vi "运维调试_采配水.vi"() -> ()   [LabVIEW 2016, in "PLC.lvlib"]
uses:
  PLC.lvlib
  <vilib>/Plasmionique/MB Master/MB_Master/MB_Master.lvclass
  <vilib>/Utility/miscctls.llb/LVPointTypeDef.ctl
  <vilib>/Plasmionique/MB Master/MB_Master_Serial/MB_Master_Serial.lvclass
  C:/Program Files (x86)/National Instruments/LabVIEW 2016/vi.lib/Plasmionique/MB Master/MB_Master/MB_Master.lvclass
  <vilib>/Plasmionique/MB Master/MB Master.lvlib
panel:
  in  "是否启用质控":u16(ring) items=["不启用质控", "启用质控"]
  out "压力传感器":dbl format="%#.2f"
  out "R110":i16 caption="过滤装置排液时间"
  out "X12":bool caption="过滤溢流液位开关"
  in  "M4":bool
  in  "M3":bool
  in  "V14NC":bool
  in  "V14NO":bool
  in  "V13NC":bool
  in  "V13NO":bool
  in  "V12":bool
  in  "V11":bool
  in  "V10":bool
  in  "V9":bool
  in  "V8":bool
  in  "V7NC":bool
  in  "V7NO":bool
  out "R113":i16 caption="反冲洗排液时间"
  out "X2":bool caption="X1"
  out "采配水版本号":string
  out "R23":i16 caption="清洗频次计数"
  out "R112":i16 caption="清洗频次设定"
  out "R111":i16 caption="排液时间"
  out "通讯故障":bool
  in  "潜水泵工作模式":u16(ring) items=["泵1单泵单管路", "泵2单泵单管路", "双泵双管路"]
  out "X11":bool caption="自来水检测"
  out "X10":bool caption="空压机压力报警"
  out "X9":bool caption="废液报警"
  out "X8":bool caption="泵2过载报警"
  out "X7":bool caption="泵1过载报警"
  out "X6":bool caption="断电检测"
  out "X5":bool caption="开门检测"
  out "X4":bool caption="烟雾检测"
  out "X3":bool caption="漏水检测"
  out "X1":bool
  out "X0":bool caption="采样池液位开关"
  out "R109":i16 caption="外部反冲洗时间"
  out "集成报警信息":string
  out "R108":i16 caption="进样超时时间"
  out "R107":i16 caption="进气时间"
  out "R106":i16 caption="反冲洗排液时间"
  out "R105":i16 caption="配水时间"
  out "R104":i16 caption="过滤次数"
  out "R103":i16 caption="过滤配水时间"
  out "R102":i16 caption="静置沉淀时间"
  out "R101":i16 caption="管路润洗时间"
  out "R100":i16 caption="外部管路润洗时间"
  out "R2":i16
  out "R1":i16
  out "多列列表框":i32(listbox)
  in  "V6":bool
  in  "V5":bool
  in  "V4":bool
  in  "V3":bool
  in  "V2":bool
  in  "M2":bool
  in  "V1":bool
  in  "M1":bool
  in  "返回":bool
  in  "参数设置":bool
  in  "单步启动":bool
  in  "启动":bool
  in  "停止":bool
  # "流程计时："
  # "s"
  # "压力传感器："
  # "MPa"
  # "二级液位开关低"
  # "二级液位开关高"
  # "次"
  # "S"
  # "S"
  # "次"
  # "次"
  # "S"
  # "S"
  # "S"
  # "S"
  # "S"
  # "S"
  # "S"
  # "S"
  # "S"
  # "单步计时："
  # "s"
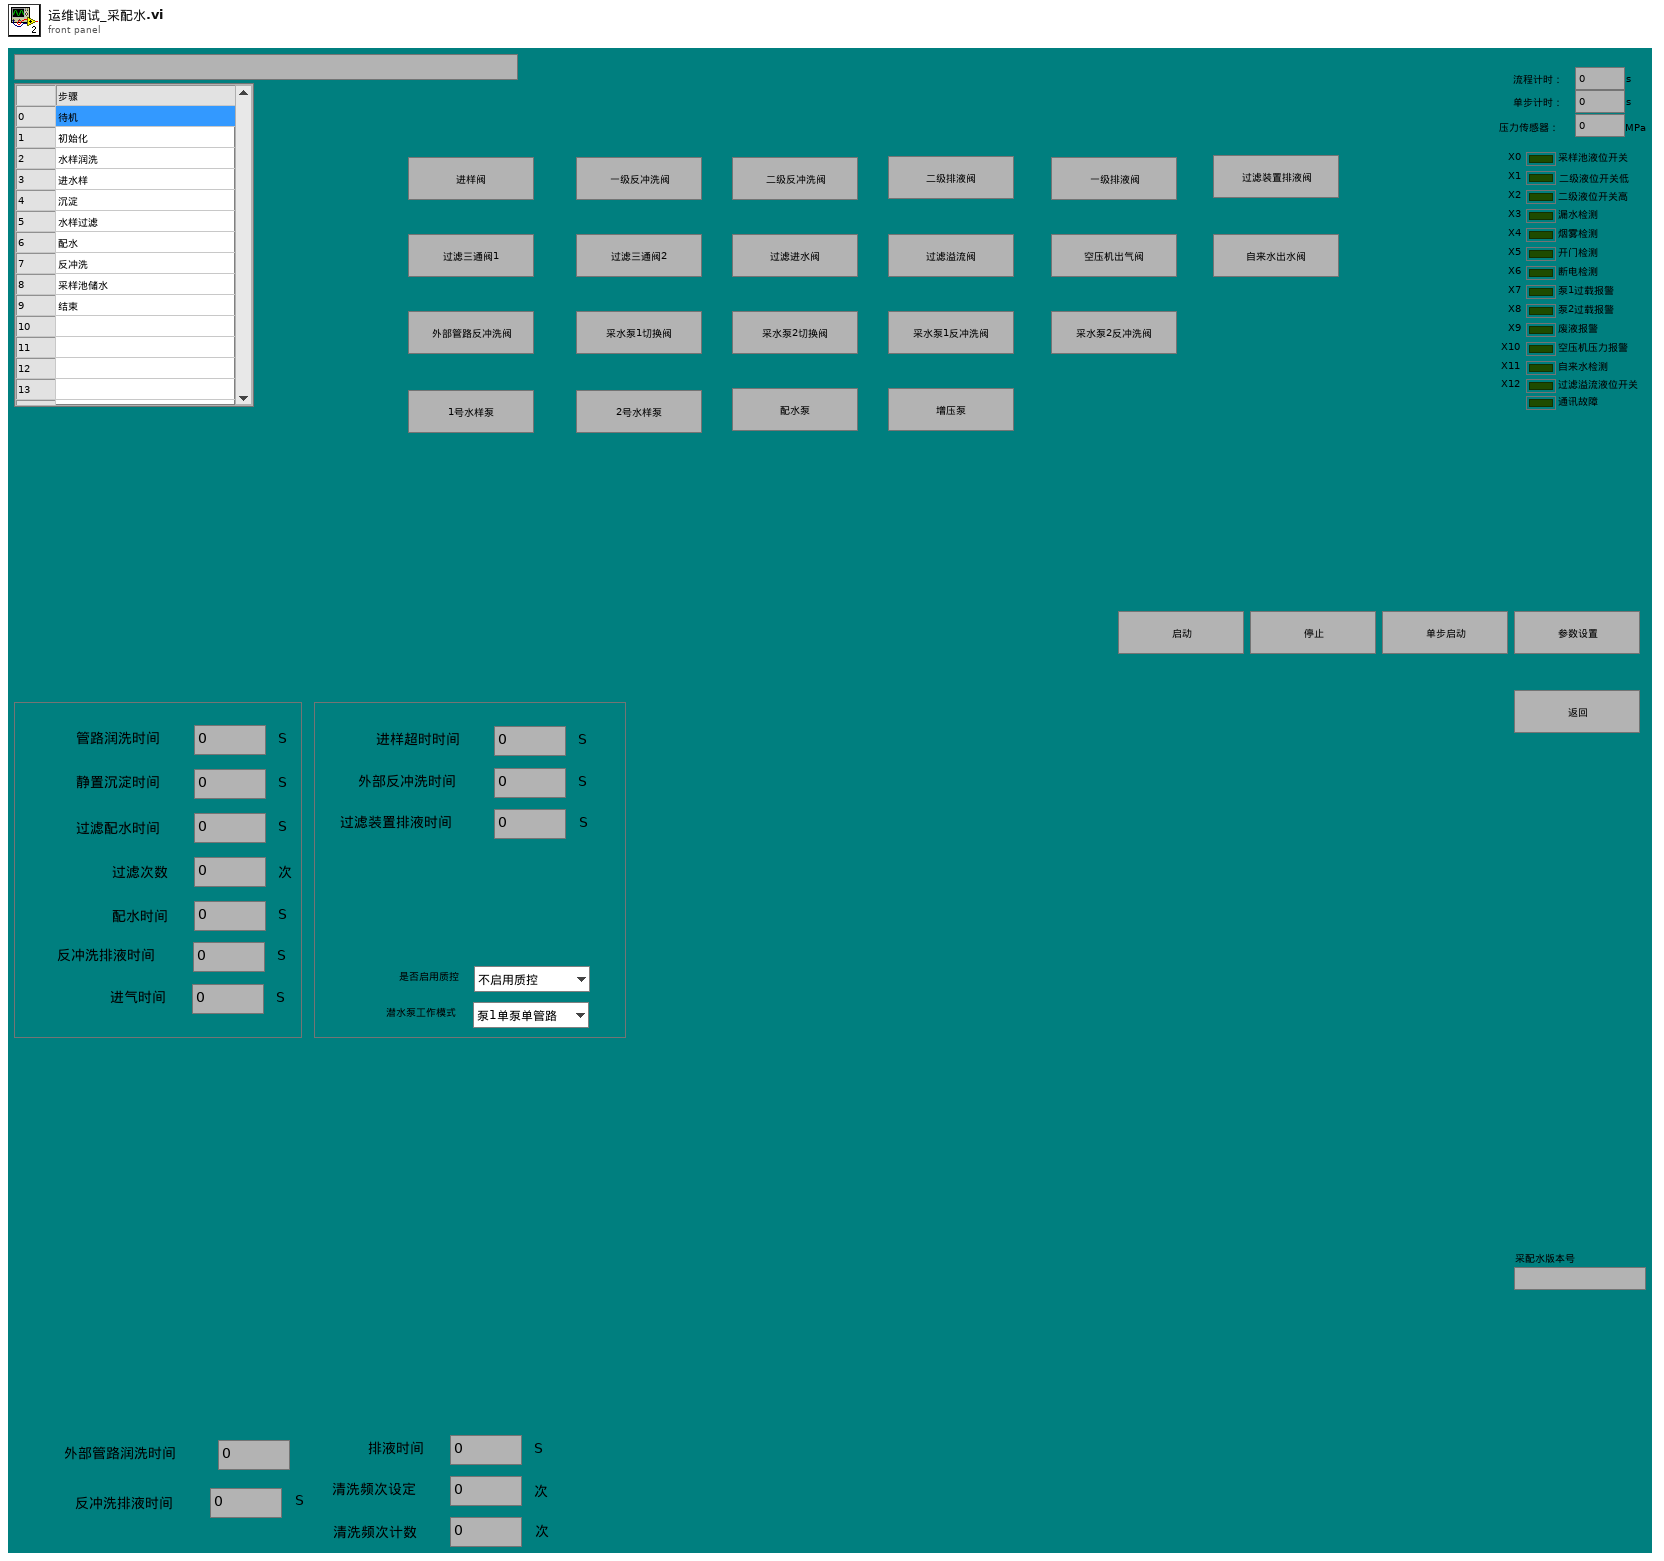
[diagram p1: front panel]
types:
  T1 = typedef "LVPointTypeDef.ctl" = cluster{"Horizontal":i16, "Vertical":i16}
  T2 = cluster{"时间标识":timestamp, "设备":string, "日志信息":string}
  T3 = cluster{"R0":i16, "R1":i16, "R2":i16, "R3":i16, "R4":i16, "R5":i16, "R6":i16, "R7":i16, "R8":i16, "R9":i16, "R10":i16, "R11":i16, "R12":i16, "R13":i16, "R14":i16, "R15":i16, "R16":i16, "R17":i16, "R18":i16, "R19":i16, "R20":i16, "R21":i16, "R22":i16, "R23":i16, "R24":i16, "R25":i16}
  T4 = cluster{"seconds since 1Jan1904":timestamp, "table输入":string, string, "table输入":string}
  T5 = cluster{"时间标识":timestamp, "设备":string, "日志信息":string, "流程参数":string}
  T6 = cluster{"命令":string, cluster{"starting address":u16, "holding register value":u16}}
  T7 = cluster{"CODCr":cluster{"启动测量模式":cluster{"测量模式":enum16{"水样测量", "标样核查", "零点核查", "加标回收", "平行样", "校零", "校标"}}, "确定按钮":bool}, "参数启用":cluster{"多参数":bool, "CODMn":bool, "总磷总氮":bool, "氨氮":bool, "CODcr":bool}}
  T8 = enum16{"水样测量", "标样核查", "零点核查", "加标回收", "平行样", "校零", "校标"}
  T9 = cluster{"命令":string, "数据":cluster{"starting address":u16, "holding register value":u16}}
  T10 = cluster{"命令":string, "数据":cluster{"starting address":u16, "holding register values":u16[]}}
  T11 = cluster{"命令":string, "data":cluster{"starting address":u16, "coil values":bool[]}}
  T12 = cluster{"多参数":bool, "CODMn":bool, "总磷总氮":bool, "氨氮":bool, "CODcr":bool}
  T13 = enum32{"Bad", "Idle", "Run top level", "Running"}
  T14 = cluster{"baud rate (bps)":u32, "stop bits":u16, "parity":u16, "flow control":u16, "timeout":u32, "retries":i32}
  T15 = cluster{"starting address":u16, "holding register values":u16[]}
  T16 = cluster{"starting address":u16, "holding register value":u16}
  T17 = cluster{"starting address":u16, "coil values":bool[]}
  T18 = cluster{"Registers[0]":u16, "Registers[1]":u16, "Registers[2]":u16, "Registers[3]":u16, "Registers[4]":u16, "Registers[5]":u16, "Registers[6]":u16, "Registers[7]":u16, "Registers[8]":u16, "Registers[9]":u16, "Registers[10]":u16, "Registers[11]":u16, "Registers[12]":u16, "Registers[13]":u16, "Registers[14]":u16, "Registers[15]":u16, "Registers[16]":u16, "Registers[17]":u16, "Registers[18]":u16, "Registers[19]":u16, "Registers[20]":u16, "Registers[21]":u16, "Registers[22]":u16, "Registers[23]":u16, "Registers[24]":u16, "Registers[25]":u16}
  T19 = cluster{"Registers[0]":u16, "Registers[1]":u16, "Registers[2]":u16, "Registers[3]":u16, "Registers[4]":u16, "Registers[5]":u16}
  T20 = cluster{"Registers[0]":u16, "Registers[1]":u16, "Registers[2]":u16, "Registers[3]":u16, "Registers[4]":u16, "Registers[5]":u16, "Registers[6]":u16, "Registers[7]":u16, "Registers[8]":u16, "Registers[9]":u16, "Registers[10]":u16, "Registers[11]":u16, "Registers[12]":u16, "Registers[13]":u16, "Registers[14]":u16, "Registers[15]":u16, "Registers[16]":u16, "Registers[17]":u16, "Registers[18]":u16, "Registers[19]":u16}
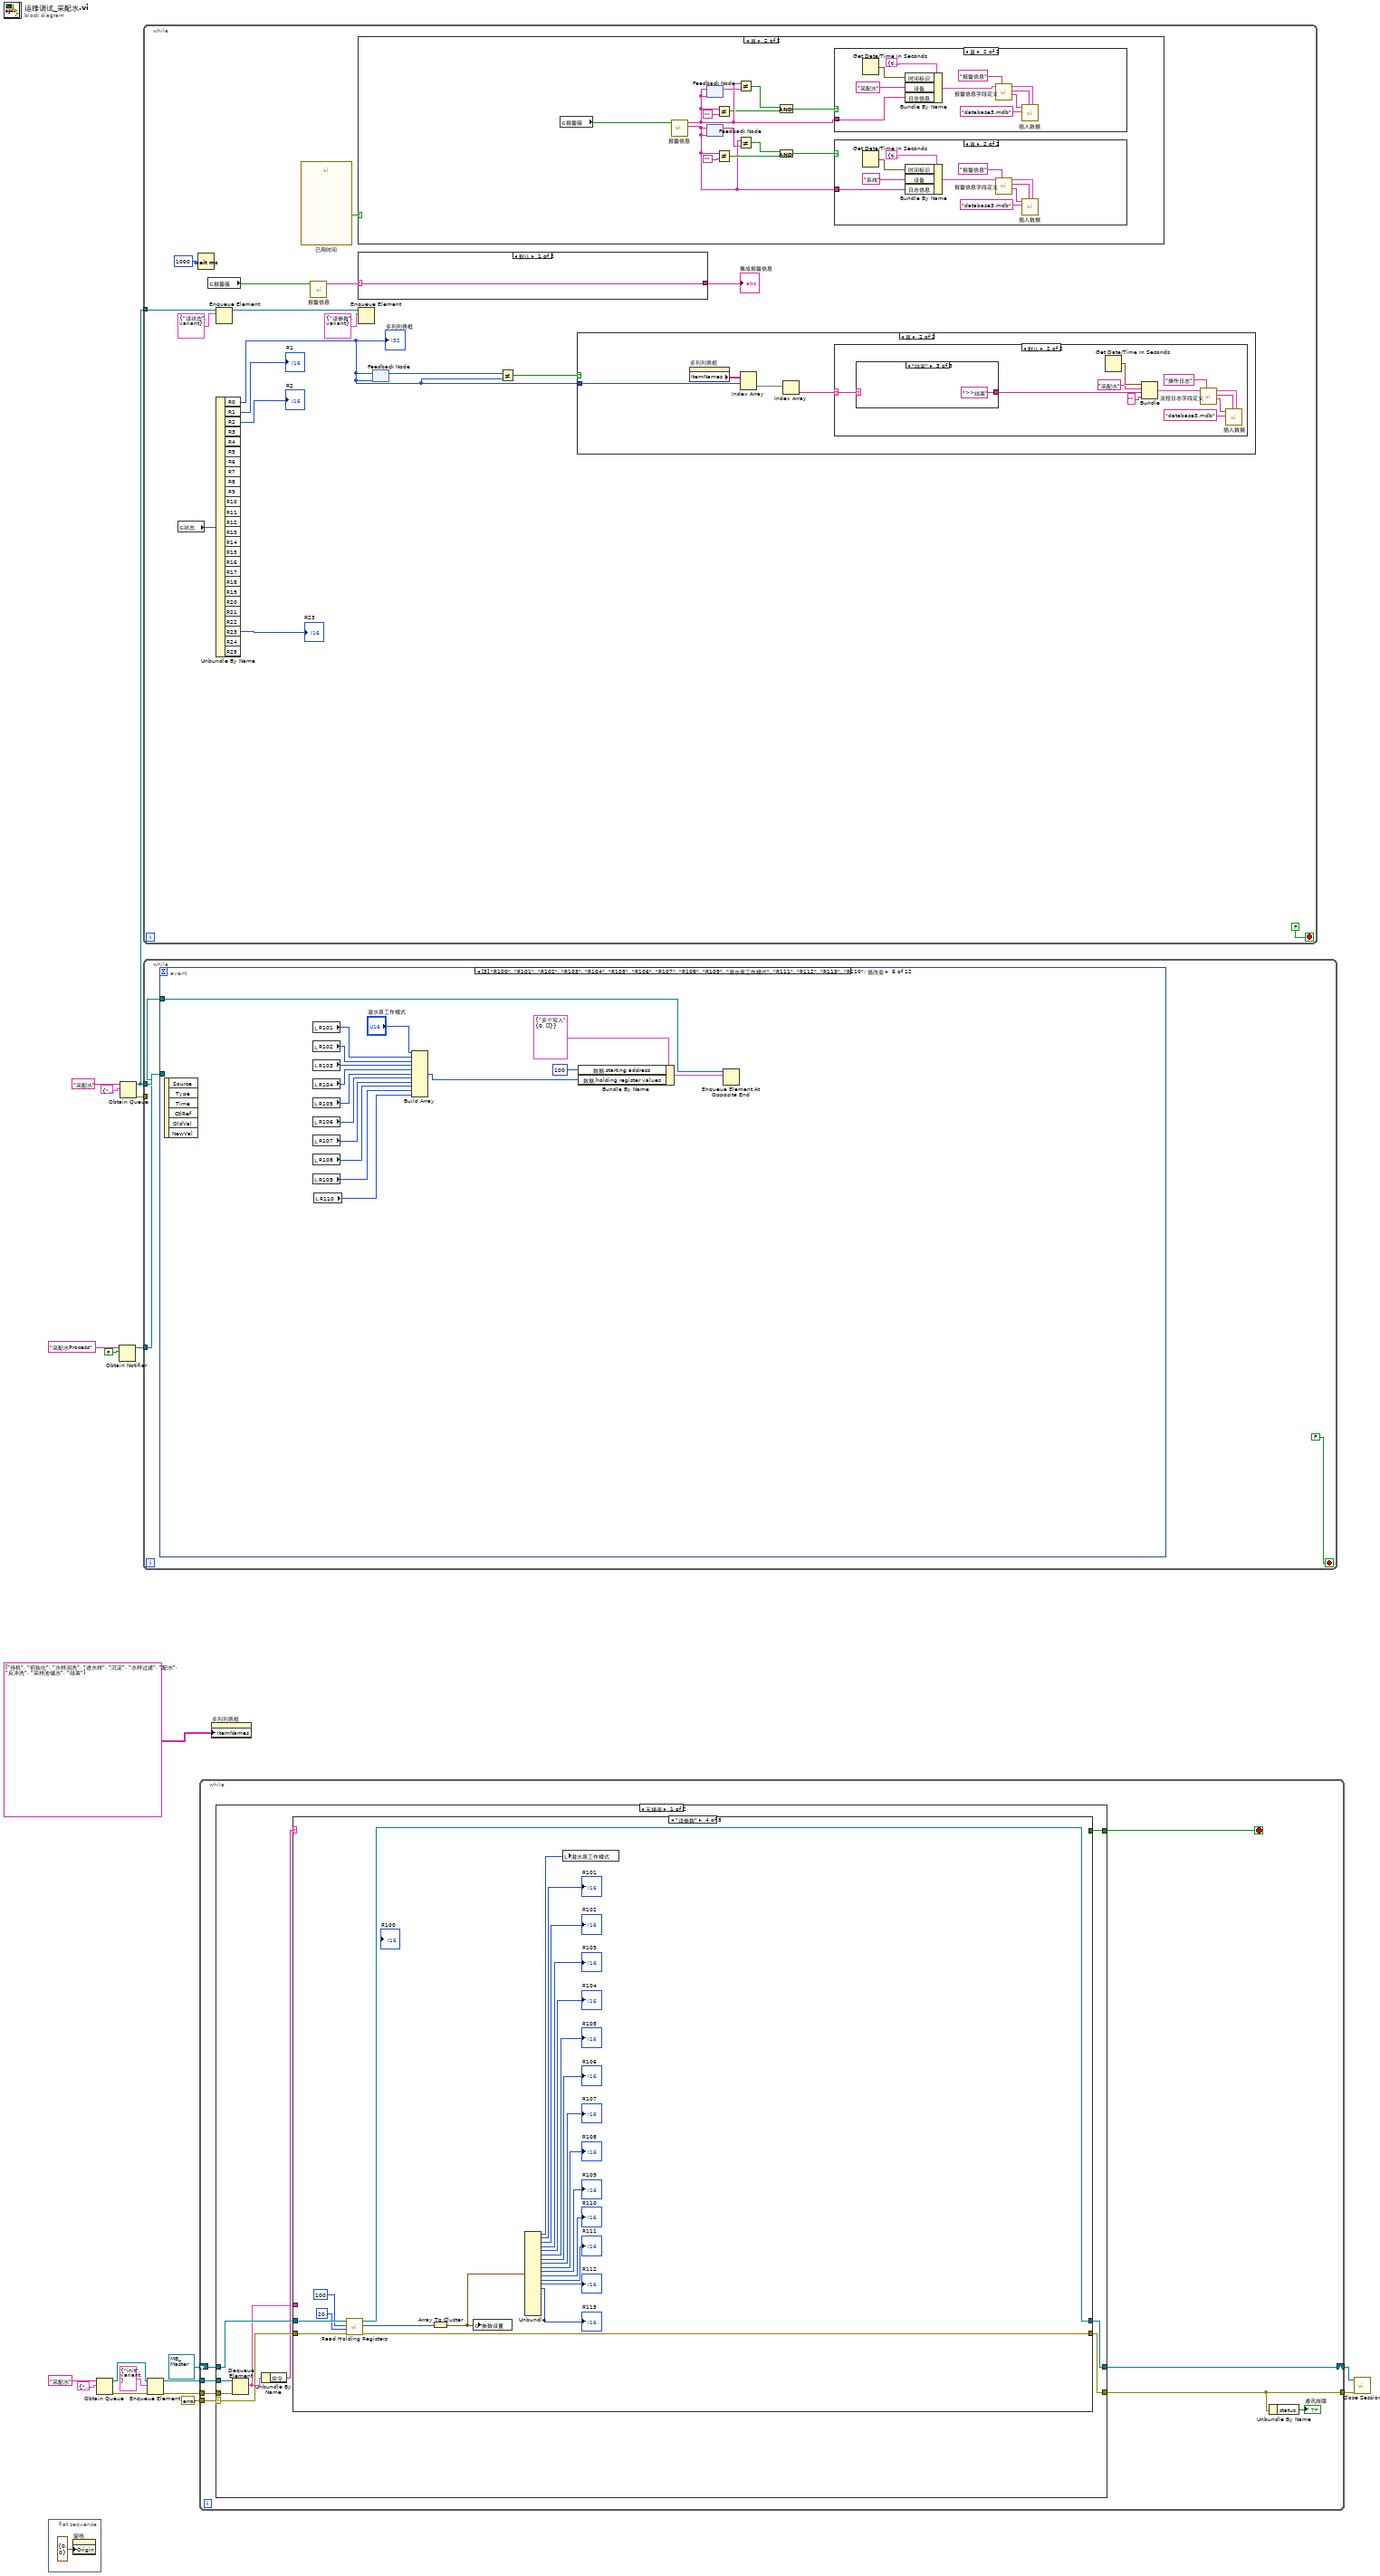
[diagram p0: block diagram]
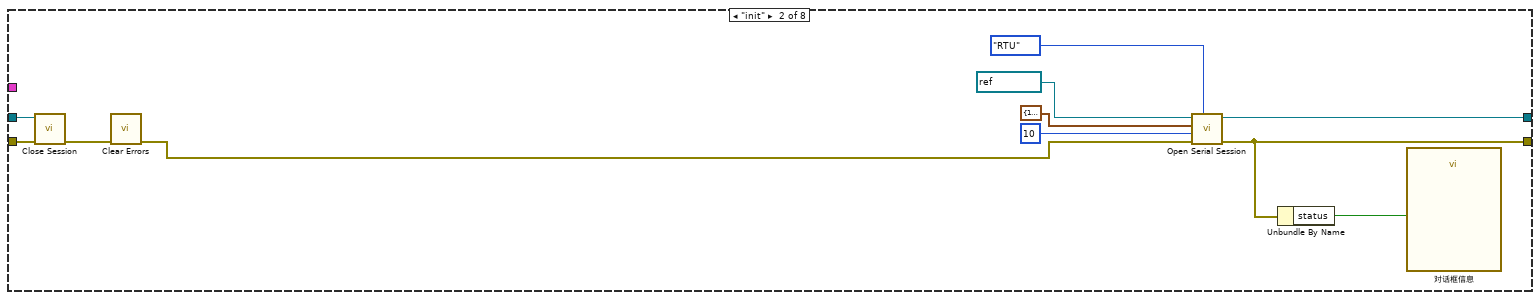
[diagram p3: hidden frame]
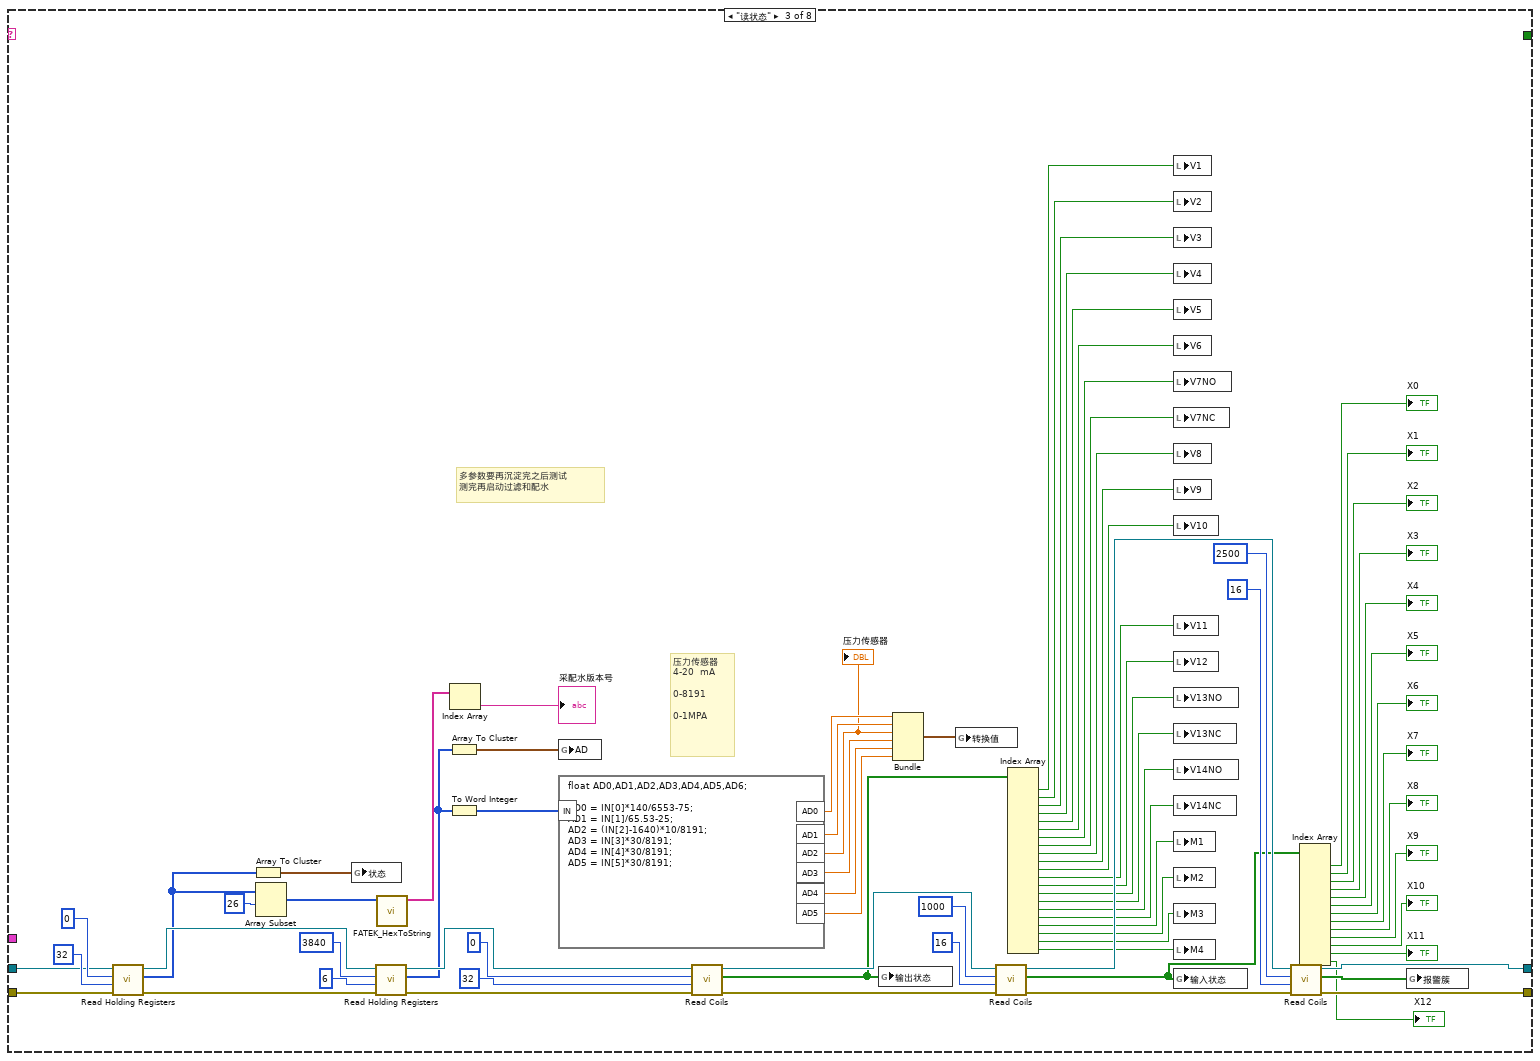
[diagram p4: hidden frame]
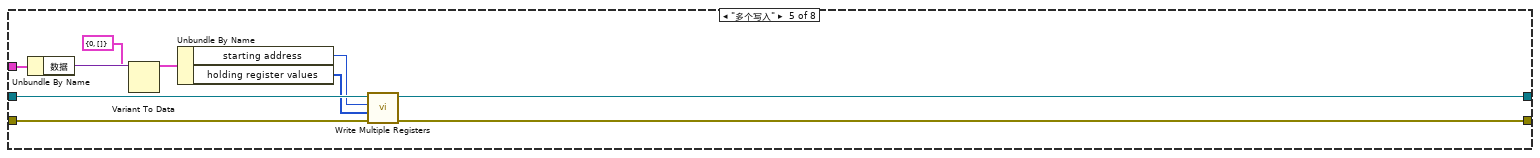
[diagram p5: hidden frame]
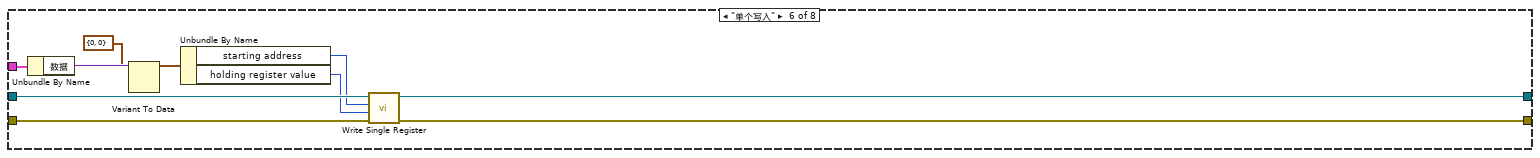
[diagram p6: hidden frame]
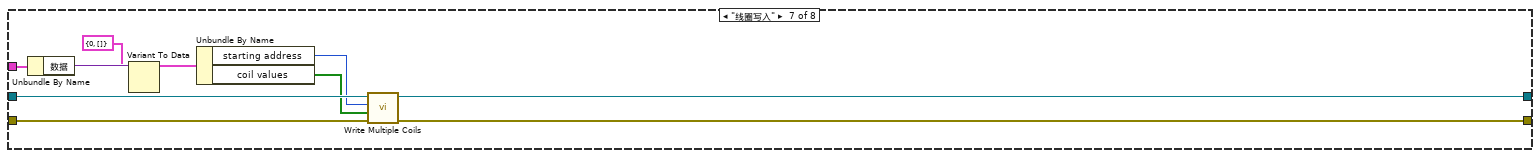
[diagram p7: hidden frame]
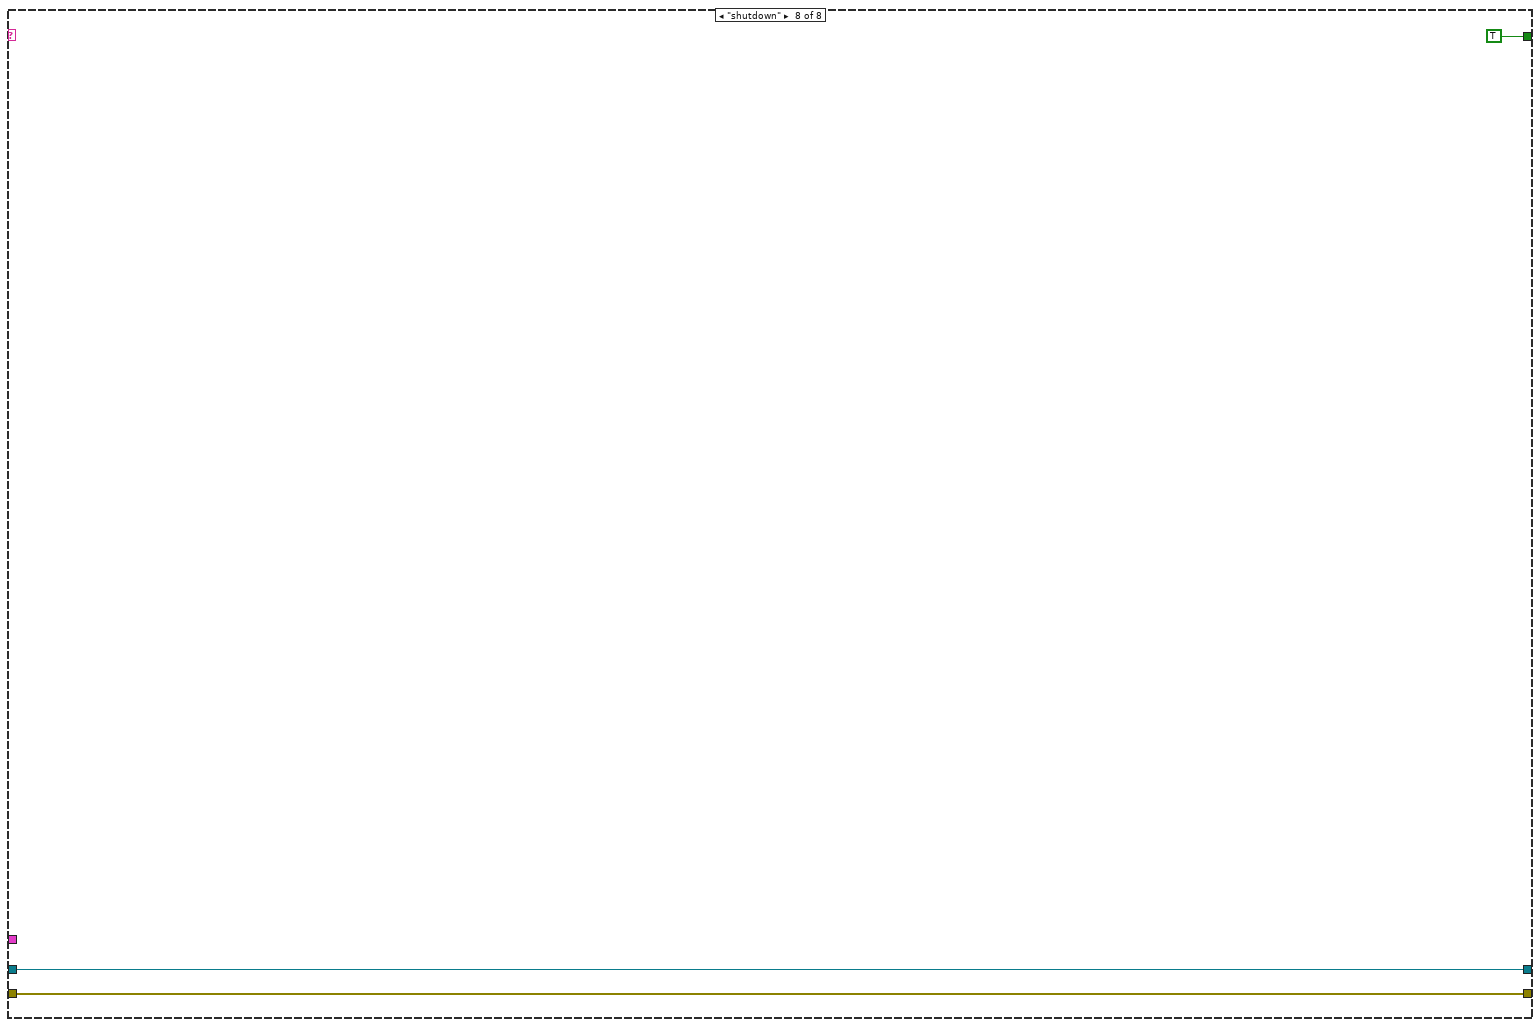
[diagram p8: hidden frame]
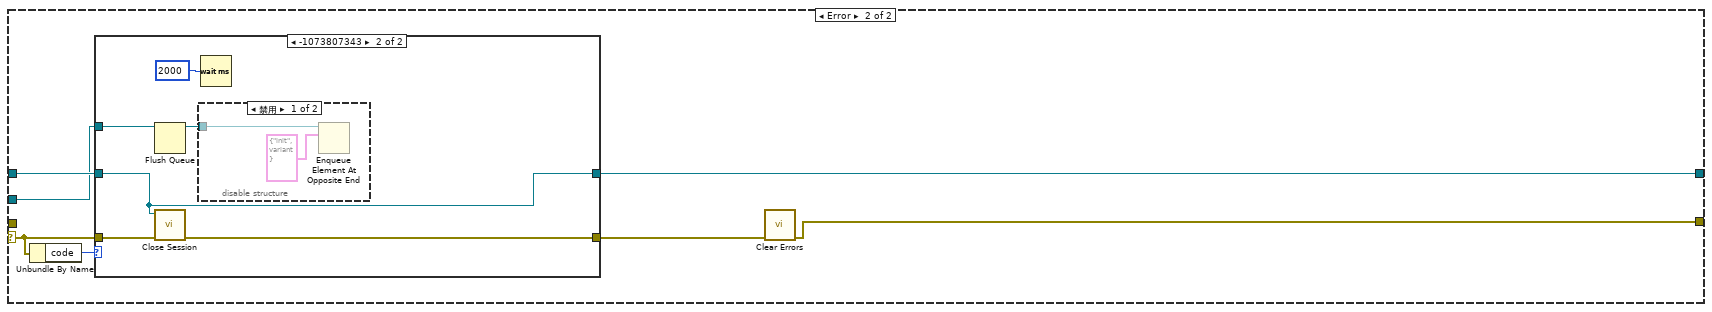
[diagram p9: hidden frame]
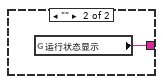
[diagram p15: hidden frame]
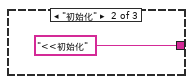
[diagram p19: hidden frame]
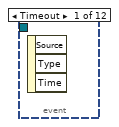
[diagram p20: hidden frame]
diagram:
  n1 = flat-sequence {
    frame #0 {
      n2 = property on="窗格" class="Pane"("Origin"=T1 {"Horizontal"=0, "Vertical"=0} ("原点")) -> ()  [unwired: 2 in, 2 out]
    }
  }
  n3 = Obtain Queue(name (unnamed)="采配水" ("名称（未命名）"), element data type=cluster{"命令":string, "数据":variant} {"命令"="", "数据"=variant}) -> (queue out=w9:refnum<queue>, error out=w8:errorcluster)  [unwired: 3 in, 1 out]
  n4 = Obtain Notifier(name (unnamed)="采配水Process" ("名称（未命名）"), notification data type=FALSE) -> (notifier out=w12:refnum<notifier>)  [unwired: 2 in, 2 out]
  n5 = Obtain Queue(name (unnamed)="采配水" ("名称（未命名）"), element data type=cluster{"命令":string, "数据":variant} {"命令"="", "数据"=variant}) -> (queue out=w16:refnum<queue>, error out=w17:errorcluster)  [unwired: 3 in, 1 out]
  n6 = while {
    tunnel: w16 -> [w36]
    stop <- FALSE stop-if-true
    n7 = global read "采配水全局变量.vi" "状态"() -> (w34:T3)
    n8 = Wait (ms)(milliseconds to wait=u32 1000 ("等待时间（毫秒）")) -> ()  [unwired: 1 out]
    n9 = global read "采配水全局变量.vi" "报警簇"() -> (w30:bool[])
    n10 = Enqueue Element(queue=w36, element=cluster{"命令":string, "数据":variant} {"命令"="读状态", "数据"=variant} ("元素")) -> (queue out=w25:refnum<queue>)  [unwired: 2 in, 2 out]
    n11 = Unbundle By Name(w34) -> ("R0"=w23:i16, "R1"=→"R1":i16, "R2"=→"R2":i16, "R23"=→"R23":i16)  [unwired: 22 out]
    "多列列表框" <- w23
    n12 = call "已用时间"() -> ("Time has Elapsed"=w28:bool)  [unwired: 12 in, 7 out]
    n13 = call "报警信息.vi"("报警簇"=w30) -> ("采配水报警信息"=w22:string)  [unwired: 9 in, 1 out]
    n14 = case shown="真" w28 {
      frame False {
      }
      frame True {
        n15 = global read "采配水全局变量.vi" "报警簇"() -> (w50:bool[])
        n16 = call "报警信息.vi"("报警簇"=w50) -> ("系统报警信息"=w39:string, "采配水报警信息"=w46:string)  [unwired: 9 in]
        n17 = feedback #1(w46) -> (w49:string)
        n18 = feedback-in #1(w46) -> ()
        n19 = feedback #2(w39) -> (w40:string)
        n20 = feedback-in #2(w39) -> ()
        n21 = Not Equal?(x=w46, y="") -> (x != y?=w44:bool)
        n22 = Not Equal?(x=w39, y="") -> (x != y?=w43:bool)
        n23 = Not Equal?(x=w46, y=w49) -> (x != y?=w48:bool)
        n24 = Not Equal?(x=w39, y=w40) -> (x != y?=w41:bool)
        n25 = And(x=w48, y=w44) -> (x .and. y?=w47:bool)
        n26 = And(x=w41, y=w43) -> (x .and. y?=w38:bool)
        n27 = case shown="真" w47 {
          tunnel: w46 -> [_ w61]
          frame False {
          }
          frame True {
            n28 = Get Date/Time In Seconds() -> (seconds since 1Jan1904=w63:timestamp)
            n29 = Bundle By Name(cluster=T2 {"时间标识"=timestamp(0 s since 1904-01-01), "设备"="", "日志信息"=""} ("data in"), "时间标识"=w63, "设备"="采配水", "日志信息"=w61) -> (w64:T2)
            n30 = call "报警信息字段定义.vi"("table输入"="报警信息", "data in"=w64) -> ("table输出"=w68:string, "columns"=w69:string[], "data out"=w70:T2)  [unwired: 7 in]
            n31 = call "插入数据.vi"("data"=w70, "columns"=w69, "database"="database3.mdb", "table"=w68) -> ()  [unwired: 7 in, 1 out]
          }
        }
        n32 = case shown="真" w38 {
          tunnel: w39 -> [_ w51]
          frame False {
          }
          frame True {
            n33 = Get Date/Time In Seconds() -> (seconds since 1Jan1904=w53:timestamp)
            n34 = Bundle By Name(cluster=T2 {"时间标识"=timestamp(0 s since 1904-01-01), "设备"="", "日志信息"=""} ("data in"), "时间标识"=w53, "设备"="系统", "日志信息"=w51) -> (w54:T2)
            n35 = call "报警信息字段定义.vi"("table输入"="报警信息", "data in"=w54) -> ("table输出"=w58:string, "columns"=w59:string[], "data out"=w60:T2)  [unwired: 7 in]
            n36 = call "插入数据.vi"("data"=w60, "columns"=w59, "database"="database3.mdb", "table"=w58) -> ()  [unwired: 7 in, 1 out]
          }
        }
      }
    }
    n37 = case shown="默认" w22 {
      selector: w22 -> [w71 _]
      tunnel: [w71 w72] -> w29
      frame Default {
      }
      frame "" {
        n38 = global read "采配水全局变量.vi" "运行状态显示"() -> (w72:string)
      }
    }
    "集成报警信息" <- w29
    n39 = Enqueue Element(queue=w25, element=cluster{"命令":string, "数据":variant} {"命令"="读参数", "数据"=variant} ("元素")) -> ()  [unwired: 2 in, 3 out]
    n40 = feedback-in #3(w23) -> ()
    n41 = feedback #3(w23) -> (w24:i16)
    n42 = Not Equal?(x=w24, y=w23) -> (x != y?=w31:bool)
    n43 = case shown="真" w31 {
      tunnel: w23 -> [_ w75]
      frame False {
      }
      frame True {
        n44 = property on="多列列表框" class="MCListbox (严格)"() -> ("ItemNames"=w76:string[][])  [unwired: 2 in, 2 out]
        n45 = Index Array(array=w76, index (row)=w75) -> (element=w74:string[])  [unwired: 1 in]
        n46 = Index Array(array=w74) -> (element=w73:string)  [unwired: 1 in]
        n47 = case shown="默认" w73 {
          selector: w73 -> [_ w78]
          frame "待机" {
          }
          frame Default {
            n48 = case shown="\"结束\"" w78 {
              selector: w78 -> [w88 _ _]
              tunnel: [w88 "<<初始化" ">>结束"] -> w77
              frame Default {
              }
              frame "初始化" {
              }
              frame "结束" {
              }
            }
            n49 = Get Date/Time In Seconds() -> (seconds since 1Jan1904=w82:timestamp)
            n50 = Bundle("seconds since 1Jan1904"=w82, "table输入"="采配水", w77, "table输入"="") -> (w80:T4)  [unwired: 1 in]
            n51 = call "流程日志字段定义.vi"("table输入"="操作日志", "data in"=w80) -> ("table输出"=w85:string, "columns"=w86:string[], "data out"=w87:T5)  [unwired: 7 in]
            n52 = call "插入数据.vi"("data"=w87, "columns"=w86, "database"="database3.mdb", "table"=w85) -> ()  [unwired: 7 in, 1 out]
          }
        }
      }
    }
  }
  n53 = while {
    tunnel: w16 -> [w92]
    tunnel: w17 -> [_]
    tunnel: w12 -> [w91]
    stop <- FALSE stop-if-true
    n54 = event shown="[5] \"R100\", \"R101\", \"R102\", \"R103\", \"R104\", \"R105\", \"R106\", \"R107\", \"R108\", \"R109\", \"潜水泵工作模式\", \"R111\", \"R112\", \"R113\", \"R110\": 值改变" {
      selector: _ -> [_ _ _ _ _ _ _ _ _ _ _ _]
      dyn-events: _ -> [_ _ _ _ _ _ _ _ _ _ _ _]
      timeout: _ -> [_ _ _ _ _ _ _ _ _ _ _ _]
      tunnel: w92 -> [_ w96 w99 w124 w128 w144 w147 _ _ _ _ w188]
      tunnel: w91 -> [_ w95 w98 _ _ _ _ _ _ _ _ _]
      event Timeout {
        n55 = event-data() -> ()  [unwired: 1 in, 3 out]
      }
      event "停止": Value Change {
        n56 = event-data() -> ()  [unwired: 1 in, 6 out]
        n57 = Send Notification(notification=TRUE ("通知"), notifier=w95) -> ()  [unwired: 1 in, 2 out]
        n58 = Enqueue Element At Opposite End(queue=w96, element=T6 {"命令"="单个写入", {"starting address"=300, "holding register value"=2}} ("元素")) -> ()  [unwired: 2 in, 3 out]
      }
      event "启动": Value Change {
        n59 = event-data() -> ()  [unwired: 1 in, 6 out]
        n60 = disable-structure shown="禁用" {
          disable-tunnel: w99 -> [w120 _]
          frame Disabled {
            n61 = Enqueue Element At Opposite End(queue=w120, element=T6 {"命令"="单个写入", {"starting address"=300, "holding register value"=1}} ("元素")) -> ()  [unwired: 2 in, 3 out]
          }
          frame Enabled {
          }
        }
        n62 = flat-sequence {
          tunnel: w98 -> [w100]
          frame #0 {
            n63 = Cancel Notification(0:w100) -> ()  [unwired: 1 in, 3 out]
          }
          frame #1 {
            n64 = call "手动启动选择对话框.vi"() -> ("确定"=w102:bool, "参数启用"=w101:T12)  [unwired: 10 in]
            n65 = case shown="真" w102 {
              tunnel: w101 -> [_ w103]
              frame False {
              }
              frame True {
                n66 = vi-ref "PLC.lvlib:一体站流程自动启动.vi"() -> (w106:refnum<vi>)
                n67 = property class="VI"(reference=w106) -> ("Name"=w105:string, "Exec.State"=w104:T13)  [unwired: 1 in, 2 out]
                n68 = case shown="\"Idle\"" w104 {
                  tunnel: w105 -> [_ w117 _ _]
                  tunnel: w103 -> [_ w107 _ _]
                  frame "Bad", Default {
                  }
                  frame "Idle" {
                    n69 = Bundle By Name(cluster=T7 {"CODCr"={"启动测量模式"={"测量模式"=enum."水样测量"}, "确定按钮"=FALSE}, "参数启用"={"多参数"=FALSE, "CODMn"=FALSE, "总磷总氮"=FALSE, "氨氮"=FALSE, "CODcr"=FALSE}} ("参数"), "CODCr.启动测量模式.测量模式"=T8."水样测量" ("CODMn.启动测量模式.测量模式"), "参数启用"=w107) -> (w108:T7)
                    n70 = Open VI Reference(type specifier VI Refnum (for type only)=refnum<vi> refnum, vi path=w117, options=128 ("选项")) -> (vi reference=w115:refnum<vi>, error out=w112:errorcluster)  [unwired: 3 in]
                    n71 = call-by-ref "开始异步调用"(reference=w115, error in=w112, "参数"=w108) -> (reference out=w113:refnum<vi>, error out=w111:errorcluster)  [unwired: 11 in]
                    n72 = Close Reference(reference=w113, error in (no error)=w111) -> ()  [unwired: 1 out]
                  }
                  frame "Run top level" {
                  }
                  frame "Running" {
                    n73 = One Button Dialog(message="流程已经运行,无须重复启动" ("消息")) -> ()  [unwired: 1 in, 1 out]
                  }
                }
              }
            }
          }
        }
      }
      event "单步启动": Value Change {
        n74 = event-data() -> ()  [unwired: 1 in, 6 out]
        n75 = call "单步启动对话框.vi"() -> ("单步启动步骤输出"=w121:u16)  [unwired: 11 in]
        n76 = Bundle By Name(cluster=T9 {"命令"="单个写入", "数据"={"starting address"=301, "holding register value"=0}} ("元素"), "数据.holding register value"=w121) -> (w122:T9)
        n77 = Enqueue Element At Opposite End(queue=w124, element=w122) -> ()  [unwired: 2 in, 3 out]
      }
      event "是否启用质控": Value Change {
        n78 = event-data() -> ()  [unwired: 1 in, 6 out]
        n79 = Bundle By Name(cluster=T9 {"命令"="单个写入", "数据"={"starting address"=120, "holding register value"=0}} ("元素"), "数据.holding register value"="是否启用质控") -> (w126:T9)
        n80 = Enqueue Element At Opposite End(queue=w128, element=w126) -> ()  [unwired: 2 in, 3 out]
      }
      event "R100", "R101", "R102", "R103", "R104", "R105", "R106", "R107", "R108", "R109", "潜水泵工作模式", "R111", "R112", "R113", "R110": Value Change {
        n81 = event-data() -> ()  [unwired: 1 in, 6 out]
        n82 = local read "R101"() -> (w140:i16)
        n83 = local read "R102"() -> (w139:i16)
        n84 = local read "R103"() -> (w138:i16)
        n85 = local read "R104"() -> (w137:i16)
        n86 = local read "R105"() -> (w136:i16)
        n87 = local read "R106"() -> (w135:i16)
        n88 = local read "R107"() -> (w134:i16)
        n89 = local read "R108"() -> (w133:i16)
        n90 = local read "R109"() -> (w131:i16)
        n91 = local read "R110"() -> (w130:i16)
        n92 = Build Array("潜水泵工作模式", w140, w139, w138, w137, w136, w135, w134, w133, w131, w130) -> (w129:u16[])
        n93 = Bundle By Name(cluster=T10 {"命令"="多个写入", "数据"={"starting address"=0, "holding register values"=[]}} ("元素"), "数据.starting address"=u16 100, "数据.holding register values"=w129) -> (w141:T10)
        n94 = Enqueue Element At Opposite End(queue=w144, element=w141) -> ()  [unwired: 2 in, 3 out]
      }
      event "R23": Value Change {
        n95 = event-data() -> ()  [unwired: 1 in, 6 out]
        n96 = local read "R23"() -> (w146:i16)
        n97 = Build Array(w146) -> (w145:i16[])
        n98 = Bundle By Name(cluster=T10 {"命令"="多个写入", "数据"={"starting address"=0, "holding register values"=[]}} ("元素"), "数据.starting address"=u16 23, "数据.holding register values"=w145) -> (w148:T10)
        n99 = Enqueue Element At Opposite End(queue=w147, element=w148) -> ()  [unwired: 2 in, 3 out]
      }
      event "R23": Mouse Down {
        n100 = event-data() -> ("CtlRef"=w153:refnum<vi>)  [unwired: 1 in, 7 out]
        n101 = Two Button Dialog(message="请确认是否更改，更改后将影响实际清洗频次" ("消息")) -> (T button?=w152:bool)  [unwired: 2 in]
        n102 = case shown="真" w152 {
          tunnel: w153 -> [_ w154]
          frame False {
          }
          frame True {
            n103 = property class="DigNum (严格)"(reference=w154) -> (reference out=w156:refnum<vi>, "Value"=w157:i16)  [unwired: 1 in, 1 out]
            n104 = call "数字键盘.vi"("OldNumber"=w157) -> ("NewNumber"=w155:sgl)
            n105 = property class="DigNum (严格)"(reference=w156, "Val(Sgnl)"=w155) -> ()  [unwired: 1 in, 2 out]
          }
        }
      }
      event "R100", "R101", "R102", "R103", "R104", "R105", "R106", "R107", "R108", "R109", "R111", "R112", "R113", "R110": Mouse Down {
        n106 = event-data() -> ("CtlRef"=w161:refnum<vi>)  [unwired: 1 in, 7 out]
        n107 = property class="DigNum (严格)"(reference=w161) -> (reference out=w159:refnum<vi>, "Value"=w160:i16)  [unwired: 1 in, 1 out]
        n108 = call "数字键盘.vi"("OldNumber"=w160) -> ("NewNumber"=w158:sgl)
        n109 = property class="DigNum (严格)"(reference=w159, "Val(Sgnl)"=w158) -> ()  [unwired: 1 in, 2 out]
      }
      event "参数设置": Value Change {
        n110 = event-data() -> ()  [unwired: 1 in, 6 out]
        n111 = property on="窗格" class="Pane"("Origin"=T1 {"Horizontal"=0, "Vertical"=628} ("原点")) -> ()  [unwired: 2 in, 2 out]
      }
      event "返回": Value Change {
        n112 = event-data() -> ()  [unwired: 1 in, 6 out]
        n113 = property on="窗格" class="Pane"("Origin"=T1 {"Horizontal"=0, "Vertical"=0} ("原点")) -> ()  [unwired: 2 in, 2 out]
      }
      event "M1", "V1", "M2", "V2", "V3", "V4", "V5", "V6", "V7NO", "V7NC", "V8", "V9", "V10", "V11", "V12", "V13NO", "V13NC", "V14NO", "V14NC", "M4", "M3": Value Change {
        n114 = event-data() -> ()  [unwired: 1 in, 6 out]
        n115 = Build Array("V1", "V2", "V3", "V4", "V5", "V6", "V7NO", "V7NC", "V8", "V9", "V10", "V11", "V12", "V13NO", "V13NC", "V14NO", "V14NC", "M1", "M2", "M3", "M4") -> (w181:bool[])
        n116 = Bundle By Name(cluster=T11 {"命令"="线圈写入", "data"={"starting address"=2400, "coil values"=[]}} ("元素"), "data.coil values"=w181) -> (w182:T11)
        n117 = Enqueue Element(queue=w188, element=w182) -> ()  [unwired: 2 in, 3 out]
      }
    }
  }
  n118 = Enqueue Element(queue=w9, element=cluster{"命令":string, "数据":variant} {"命令"="init", "数据"=variant} ("元素"), error in (no error)=w8) -> (queue out=w4:refnum<queue>, error out=w6:errorcluster)  [unwired: 1 in, 1 out]
  n119 = while {
    tunnel: w4 -> [w193]
    tunnel: w6 -> [w192]
    shift-right: [w196] -> w1
    shift-left: refnum<class "MB_Master.lvclass"> refnum ("MB session in") -> [w195]
    tunnel: errorcluster {"status"=FALSE, "code"=0, "source"=""} ("error out") -> [w194]
    tunnel: [w190] -> w2
    stop <- w191 stop-if-true
    n120 = case shown="无错误" w194 {
      selector: w194 -> [w202 w353]
      tunnel: [w205 w352] -> w196
      tunnel: w195 -> [w204 w354]
      tunnel: [w203 w350] -> w190
      tunnel: w193 -> [w199 w349]
      tunnel: w192 -> [w198 _]
      tunnel: [w200 _] -> w191
      frame No Error {
        n121 = Dequeue Element(queue=w199, error in (no error)=w198) -> (element=w197:cluster{"命令":string, "数据":variant})  [unwired: 1 in, 3 out]
        n122 = Unbundle By Name(w197) -> ("命令"=w201:string)
        n123 = case shown="\"读参数\"" w201 {
          tunnel: [w207 w211 w264 w310 w322 w332 w342 w347] -> w205
          tunnel: w204 -> [w207 w215 w282 w315 w325 w335 w345 w347]
          tunnel: [w206 w213 w263 w309 w323 w333 w343 w346] -> w203
          tunnel: w202 -> [w206 w217 w285 w314 w324 w334 w344 w346]
          tunnel: [_ _ _ _ _ _ _ TRUE] -> w200
          tunnel: w197 -> [_ _ _ _ w321 w331 w341 _]
          frame "idle", Default {
          }
          frame "init" {
            n124 = call-dynamic "Close Session.vi"("error in (no error)"=w217, "MB session in"=w215) -> ("error out"=w216:errorcluster)  [unwired: 9 in]
            n125 = call <vilib>:"Clear Errors.vi"("error in (no error)"=w216) -> ("error out"=w214:errorcluster)  [unwired: 5 in, 1 out]
            n126 = call <vilib>:"Open Serial Session.vi"("Mode (RTU)"=enum16{"RTU", "ASCII"}."RTU", "Error in"=w214, "Slave ID"=u8 10, "Serial Config"=T14 {"baud rate (bps)"=115200, "stop bits"=10, "parity"=0, "flow control"=0, "timeout"=500, "retries"=1}, "VISA Resource"=refnum<visa-resource-name> "COM3" ("VISA resource name")) -> ("Error out"=w213:errorcluster, "MB_Serial session"=w211:refnum<class "MB_Master_Serial.lvclass">)  [unwired: 5 in]
            n127 = Unbundle By Name(w213) -> ("status"=w218:bool)
            n128 = call "对话框信息"("Enable"=w218) -> ()  [unwired: 9 in, 2 out]
          }
          frame "读状态" {
            # "多参数要再沉淀完之后测试\n测完再启动过滤和配水"
            # "压力传感器\n4-20  mA \n \n0-8191\n\n0-1MPA"
            n129 = call <vilib>:"Read Holding Registers.vi"("error in (no error)"=w285, "quantity"=u16 32 ("number of holding registers"), "starting address"=u16 0, "MB session in"=w282) -> ("error out"=w280:errorcluster, "Registers"=w249:u16[], "MB session out"=w281:refnum<class "MB_Master.lvclass">)  [unwired: 5 in]
            n130 = Array To Cluster(array=w249) -> (cluster=w286:T18)
            n131 = Array Subset(array=w249, index=26 ("索引")) -> (w247:u16[])  [unwired: 1 in]
            n132 = global write "采配水全局变量.vi" "状态"(w286) -> ()
            n133 = call <vilib>:"Read Holding Registers.vi"("error in (no error)"=w280, "quantity"=u16 6 ("number of holding registers"), "starting address"=u16 3840, "MB session in"=w281) -> ("error out"=w276:errorcluster, "Registers"=w251:u16[], "MB session out"=w277:refnum<class "MB_Master.lvclass">)  [unwired: 5 in]
            n134 = call "FATEK_HexToString.vi"("数组"=w247) -> ("STRING"=w246:string[])  [unwired: 10 in]
            n135 = Array To Cluster(array=w251) -> (cluster=w293:T19)
            n136 = To Word Integer(number=w251) -> (16bit integer=w250:i16[])
            n137 = Index Array(array=w246) -> (element=→"采配水版本号":string)  [unwired: 1 in]
            n138 = global write "采配水全局变量.vi" "AD"(w293) -> ()
            n139 = formula code="float AD0,AD1,AD2,AD3,AD4,AD5,AD6;\n\nAD0 = IN[0]*140/6553-75;\nAD1 = IN[1]/65.53-25;\nAD2 = (IN[2]-1640)*10/8191;\nAD3 = IN[3]*30/8191;\nAD4 = IN[4]*30/8191;\nAD5 = IN[5]*30/8191;"("IN"=w250) -> ("AD0"=w291:dbl, "AD1"=w290:dbl, "AD2"=w220:dbl, "AD3"=w289:dbl, "AD4"=w288:dbl, "AD5"=w287:dbl)
            "压力传感器" <- w220
            n140 = call <vilib>:"Read Coils.vi"("error in (no error)"=w276, "quantity"=u16 32 ("number of coils"), "starting address"=u16 0, "MB session in"=w277) -> ("error out"=w272:errorcluster, "Coils"=w255:bool[], "MB session out"=w273:refnum<class "MB_Master.lvclass">)  [unwired: 5 in]
            n141 = global write "采配水全局变量.vi" "输出状态"(w255) -> ()
            n142 = Bundle(w291, w290, w220, w289, w288, w287) -> (w292:cluster{dbl, dbl, dbl, dbl, dbl, dbl})  [unwired: 1 in]
            n143 = global write "采配水全局变量.vi" "转换值"(w292) -> ()
            n144 = call <vilib>:"Read Coils.vi"("error in (no error)"=w272, "quantity"=u16 16 ("number of coils"), "starting address"=u16 1000, "MB session in"=w273) -> ("error out"=w268:errorcluster, "Coils"=w262:bool[], "MB session out"=w269:refnum<class "MB_Master.lvclass">)  [unwired: 5 in]
            n145 = Index Array(array=w255) -> (element #1=w244:bool, element #2=w243:bool, element #3=w242:bool, element #4=w241:bool, element #5=w240:bool, element #6=w239:bool, element #7=w235:bool, element #8=w234:bool, element #9=w233:bool, element #10=w232:bool, element #11=w231:bool, element #12=w230:bool, element #13=w229:bool, element #14=w228:bool, element #15=w227:bool, element #16=w226:bool, element #17=w225:bool, element #18=w224:bool, element #19=w223:bool, element #20=w222:bool, element #21=w221:bool)  [unwired: 21 in]
            n146 = local write "V1"(w244) -> ()
            n147 = local write "V2"(w243) -> ()
            n148 = local write "V3"(w242) -> ()
            n149 = local write "V4"(w241) -> ()
            n150 = local write "V5"(w240) -> ()
            n151 = local write "V6"(w239) -> ()
            n152 = local write "V7NO"(w235) -> ()
            n153 = local write "V7NC"(w234) -> ()
            n154 = local write "V8"(w233) -> ()
            n155 = local write "V9"(w232) -> ()
            n156 = local write "V10"(w231) -> ()
            n157 = local write "V11"(w230) -> ()
            n158 = local write "V12"(w229) -> ()
            n159 = local write "V13NO"(w228) -> ()
            n160 = local write "V13NC"(w227) -> ()
            n161 = local write "V14NO"(w226) -> ()
            n162 = local write "V14NC"(w225) -> ()
            n163 = local write "M1"(w224) -> ()
            n164 = local write "M2"(w223) -> ()
            n165 = local write "M3"(w222) -> ()
            n166 = local write "M4"(w221) -> ()
            n167 = global write "采配水全局变量.vi" "输入状态"(w262) -> ()
            n168 = call <vilib>:"Read Coils.vi"("error in (no error)"=w268, "quantity"=u16 16 ("number of coils"), "starting address"=u16 2500, "MB session in"=w269) -> ("error out"=w263:errorcluster, "Coils"=w265:bool[], "MB session out"=w264:refnum<class "MB_Master.lvclass">)  [unwired: 5 in]
            n169 = Index Array(array=w262) -> (element #1=→"X0":bool, element #2=→"X1":bool, element #3=→"X2":bool, element #4=→"X3":bool, element #5=→"X4":bool, element #6=→"X5":bool, element #7=→"X6":bool, element #8=→"X7":bool, element #9=→"X8":bool, element #10=→"X9":bool, element #11=→"X10":bool, element #12=→"X11":bool, element #13=→"X12":bool)  [unwired: 13 in]
            n170 = global write "采配水全局变量.vi" "报警簇"(w265) -> ()
          }
          frame "读参数" {
            n171 = call <vilib>:"Read Holding Registers.vi"("error in (no error)"=w314, "quantity"=u16 20 ("number of holding registers"), "starting address"=u16 100, "MB session in"=w315) -> ("error out"=w309:errorcluster, "Registers"=w311:u16[], "MB session out"=w310:refnum<class "MB_Master.lvclass">)  [unwired: 5 in]
            n172 = Array To Cluster(array=w311) -> (cluster=w299:T20)
            n173 = global write "采配水全局变量.vi" "参数设置"(w299) -> ()
            n174 = Unbundle(w299) -> ("Registers[0]"=w295:u16, "Registers[1]"=→"R101":u16, "Registers[2]"=→"R102":u16, "Registers[3]"=→"R103":u16, "Registers[4]"=→"R104":u16, "Registers[5]"=→"R105":u16, "Registers[6]"=→"R106":u16, "Registers[7]"=→"R107":u16, "Registers[8]"=→"R108":u16, "Registers[9]"=→"R109":u16, "Registers[10]"=→"R110":u16, "Registers[11]"=→"R111":u16, "Registers[12]"=→"R112":u16, "Registers[13]"=→"R113":u16)  [unwired: 6 out]
            n175 = local write "潜水泵工作模式"(w295) -> ()
          }
          frame "多个写入" {
            n176 = Unbundle By Name(w321) -> ("数据"=w320:variant)
            n177 = Variant To Data(type=T15 {"starting address"=0, "holding register values"=[]}, Variant=w320) -> (data=w318:T15)  [unwired: 1 in, 1 out]
            n178 = Unbundle By Name(w318) -> ("starting address"=w317:u16, "holding register values"=w316:u16[])
            n179 = call <vilib>:"Write Multiple Registers.vi"("error in (no error)"=w324, "values"=w316, "starting address"=w317, "MB session in"=w325) -> ("error out"=w323:errorcluster, "MB session out"=w322:refnum<class "MB_Master.lvclass">)  [unwired: 6 in]
          }
          frame "单个写入" {
            n180 = Unbundle By Name(w331) -> ("数据"=w330:variant)
            n181 = Variant To Data(type=T16 {"starting address"=0, "holding register value"=0}, Variant=w330) -> (data=w328:T16)  [unwired: 1 in, 1 out]
            n182 = Unbundle By Name(w328) -> ("starting address"=w327:u16, "holding register value"=w326:u16)
            n183 = call <vilib>:"Write Single Register.vi"("error in (no error)"=w334, "value"=w326, "address"=w327, "MB session in"=w335) -> ("error out"=w333:errorcluster, "MB session out"=w332:refnum<class "MB_Master.lvclass">)  [unwired: 6 in]
          }
          frame "线圈写入" {
            n184 = Unbundle By Name(w341) -> ("数据"=w340:variant)
            n185 = Variant To Data(type=T17 {"starting address"=0, "coil values"=[]}, Variant=w340) -> (data=w338:T17)  [unwired: 1 in, 1 out]
            n186 = Unbundle By Name(w338) -> ("starting address"=w337:u16, "coil values"=w336:bool[])
            n187 = call <vilib>:"Write Multiple Coils.vi"("error in (no error)"=w344, "values"=w336, "starting address"=w337, "MB session in"=w345) -> ("error out"=w343:errorcluster, "MB session out"=w342:refnum<class "MB_Master.lvclass">)  [unwired: 6 in]
          }
          frame "shutdown" {
          }
        }
      }
      frame Error {
        n188 = Unbundle By Name(w353) -> ("code"=w355:i32)
        n189 = case shown="-1073807343" w355 {
          tunnel: w354 -> [w357 w361]
          tunnel: w353 -> [w356 w363]
          tunnel: [w356 w362] -> w351
          tunnel: [w357 w361] -> w352
          tunnel: w349 -> [_ w360]
          frame Default {
          }
          frame -1073807343 {
            n190 = Flush Queue(queue=w360) -> (queue out=w359:refnum<queue>)  [unwired: 1 in, 2 out]
            n191 = call-dynamic "Close Session.vi"("error in (no error)"=w363, "MB session in"=w361) -> ("error out"=w362:errorcluster)  [unwired: 9 in]
            n192 = disable-structure shown="禁用" {
              disable-tunnel: w359 -> [w364 _]
              frame Disabled {
                n193 = Enqueue Element At Opposite End(queue=w364, element=cluster{"命令":string, "数据":variant} {"命令"="init", "数据"=variant} ("元素")) -> ()  [unwired: 2 in, 3 out]
              }
              frame Enabled {
              }
            }
            n194 = Wait (ms)(milliseconds to wait=u32 2000 ("等待时间（毫秒）")) -> ()  [unwired: 1 out]
          }
        }
        n195 = call <vilib>:"Clear Errors.vi"("error in (no error)"=w351) -> ("error out"=w350:errorcluster)  [unwired: 5 in, 1 out]
      }
    }
    n196 = Unbundle By Name(w190) -> ("status"=→"通讯故障":bool)
  }
  n197 = property on="多列列表框" class="MCListbox (严格)"("ItemNames"=string[][] [["待机"], ["初始化"], ["水样润洗"], ["进水样"], ["沉淀"], ["水样过滤"], ["配水"], ["反冲洗"], ["采样池储水"], ["结束"]] ("项名")) -> ()  [unwired: 2 in, 2 out]
  n198 = call-dynamic "Close Session.vi"("error in (no error)"=w2, "MB session in"=w1) -> ()  [unwired: 9 in, 1 out]
